vi "HIL.vi"(2 "U":dbl[](array[numeric])) -> (10 "eta":dbl[](array[numeric]))   [LabVIEW 2014]
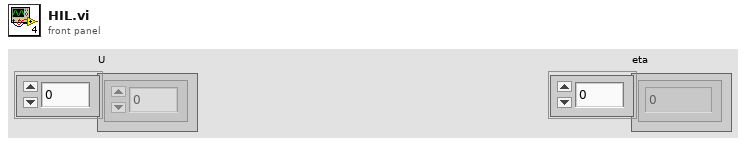
[diagram p1: front panel]
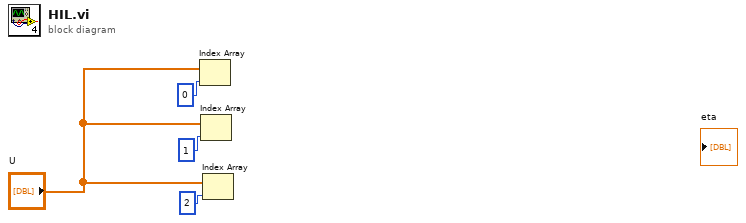
[diagram p0: block diagram]
diagram:
  n1 = Index Array(array="U", index=0) -> ()  [unwired: 1 out]
  n2 = Index Array(array="U", index=1) -> ()  [unwired: 1 out]
  n3 = Index Array(array="U", index=2) -> ()  [unwired: 1 out]
